vi "GetName.vi"(6 "error in":errorcluster, 9 "Tunnel in":refnum<class "FlatSequenceOuterTunnel.lvclass">) -> (0 "error out":errorcluster, 3 "Tunnel out":refnum<class "FlatSequenceOuterTunnel.lvclass">, 4 "name":string)   [LabVIEW 2014, in "Raspberry Pi Compatible Compiler for LabVIEW.lvlib" / "FlatSequenceOuterTunnel.lvclass"]
uses:
  FlatSequenceOuterTunnel.lvclass
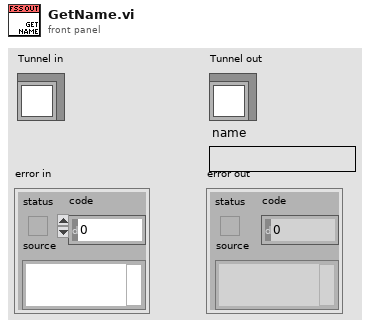
[diagram p1: front panel]
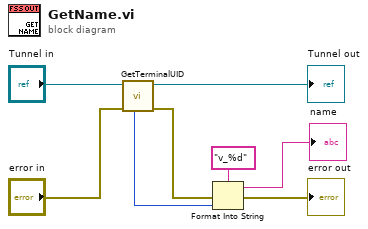
[diagram p0: block diagram]
diagram:
  n1 = call "GetTerminalUID.vi"("error in"="error in", "Tunnel in"="Tunnel in") -> ("error out"=w4:errorcluster, "Tunnel out"=→"Tunnel out":refnum<class "FlatSequenceOuterTunnel.lvclass">, "inside terminal UID"=w1:i32)  [unwired: 4 in, 1 out]
  n2 = Format Into String(format string="v_%d", error in=w4, w1) -> (resulting string=→"name":string, error out=→"error out":errorcluster)  [unwired: 1 in]
